vi "Voltage Read.vi"   [LabVIEW 2023, in "Cycler.lvclass"]
uses:
  Cycler.lvclass
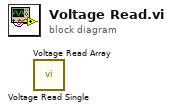
[diagram p0: block diagram]
diagram:
  n1 = call "Voltage Read Single.vi"() -> ()  [unwired: 8 in, 4 out]
  n2 = call "Voltage Read Array.vi"() -> ()  [unwired: 9 in, 3 out]
